vi "setState.vi"(0 "Interface in":T2, 7 "state":T1, 11 "error in (no error)":errorcluster) -> (4 "Interface out":T2, 15 "error out":errorcluster)   [LabVIEW 2017, in "BuckBoostInterface.lvlib"]
uses:
  BuckBoostInterface.lvlib
  Interface.ctl
  <instrlib>/_niInstr/Instruction Framework/v1/Host/Instruction Target/niInstr Instruction Target v1 Host.lvclass
  <instrlib>/_niInstr/Instruction Framework/v1/Host/Instruction Framework Context/niInstr Instruction Framework Context v1 Host.lvclass
  FPGA/contState.ctl
  <vilib>/NI/JSON Support for LabVIEW/JSON Data Classes/JSON Object/New JSON Object (Empty).vi
  <vilib>/NI/JSON Support for LabVIEW/JSON Data Classes/JSON Object/Insert Key Value Pair (Single).vi
  <vilib>/NI/JSON Support for LabVIEW/JSON Data Classes/JSON Helper/Parsing/Parse Value.vi
  <vilib>/NI/JSON Support for LabVIEW/JSON Data Classes/JSON Helper/To More Specific Type (Object).vi
  <vilib>/NI/JSON Support for LabVIEW/JSON Data Classes/JSON Datatype/JSON Null.lvclass
  <vilib>/NI/JSON Support for LabVIEW/JSON Data Classes/JSON Object/JSON Object.lvclass
  <vilib>/NI/JSON Support for LabVIEW/JSON Data Classes/JSON Helper/JSON Helper.lvclass
  FPGA/BuckBoost.lvlib
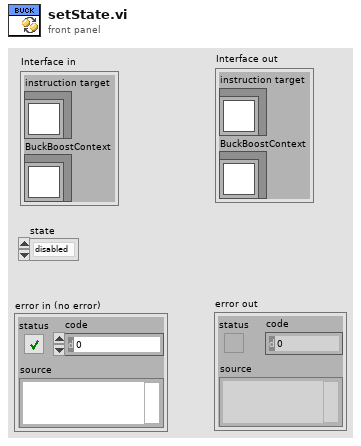
[diagram p1: front panel]
types:
  T1 = typedef "BuckBoost.lvlib/contState.ctl" = enum16{"disabled", "manual", "normal", "perturb"}
  T2 = typedef "BuckBoostInterface.lvlib/Interface.ctl" = cluster{"instruction target":refnum<class "niInstr Instruction Target v1 Host.lvclass">, "BuckBoostContext":refnum<class "niInstr Instruction Framework Context v1 Host.lvclass">}
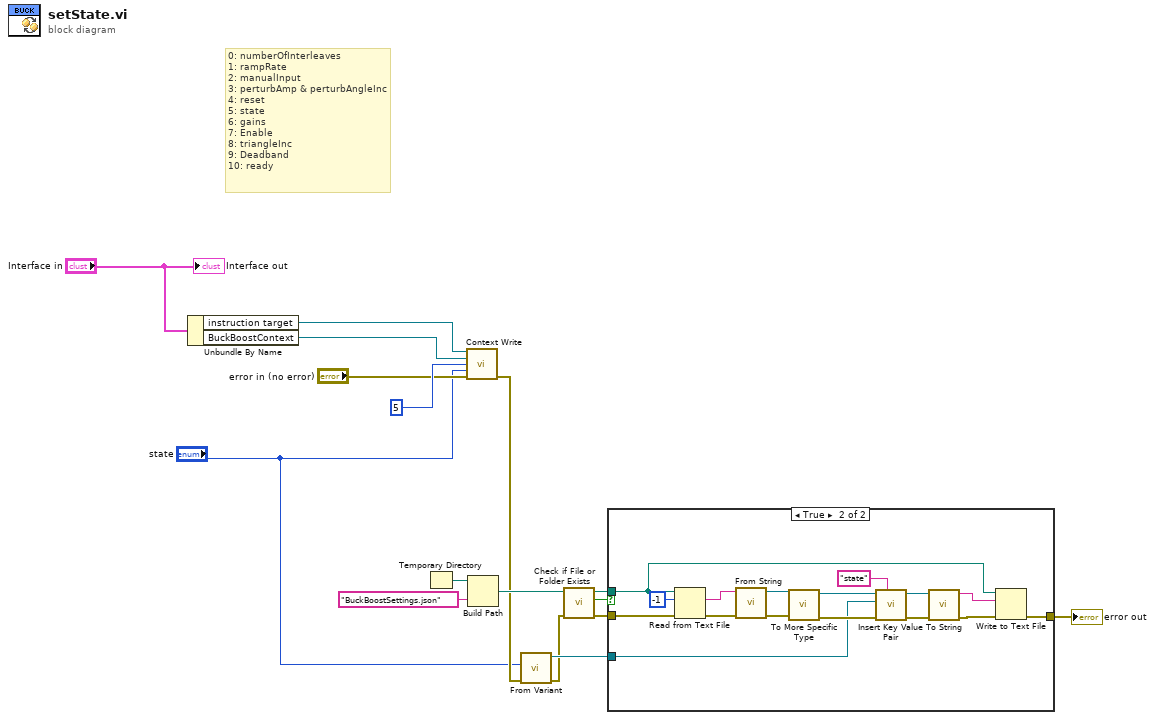
[diagram p0: block diagram]
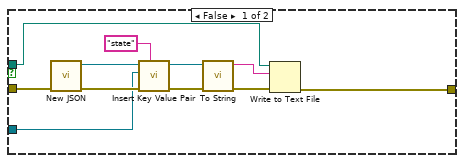
[diagram p2: hidden frame]
diagram:
  # "0: numberOfInterleaves\n1: rampRate\n2: manualInput\n3: perturbAmp & perturbAngleInc\n4: reset\n5: state\n6: gains\n7: Enable\n8: triangleInc\n9: Deadband\n10: ready"
  n1 = Unbundle By Name("Interface in") -> ("instruction target"=w13:refnum<class "niInstr Instruction Target v1 Host.lvclass">, "BuckBoostContext"=w12:refnum<class "niInstr Instruction Framework Context v1 Host.lvclass">)
  n2 = Temporary Directory() -> (w11:path)
  n3 = call <instrlib>:"Context Write.vi"("instruction target in"=w13, "context in"=w12, "address"=u64 5, "data"="state", "error in"="error in (no error)") -> ("error out"=w3:errorcluster)  [unwired: 8 in, 2 out]
  n4 = Build Path(base path=w11, name or relative path="BuckBoostSettings.json") -> (appended path=w9:path)
  n5 = call <vilib>:"From Variant.vi"("error in (no error)"=w3, "Variant"="state") -> ("error out"=w4:errorcluster, "JSON out"=w6:refnum<class "JSON Null.lvclass">)  [unwired: 8 in]
  n6 = call <vilib>:"Check if File or Folder Exists.vi"("error in (no error)"=w4, "path"=w9) -> ("error out"=w5:errorcluster, "file or folder exists?"=w7:bool, "dup path"=w8:path)  [unwired: 7 in]
  n7 = case shown="True" w7 {
    tunnel: w8 -> [w22 w34]
    tunnel: w6 -> [w24 w36]
    tunnel: w5 -> [w27 w35]
    tunnel: [w21 w29] -> w2
    frame False {
      n8 = call-poly <vilib>:"New JSON.vi"("error in (no error)"=w27) -> ("error out"=w25:errorcluster, "JSON Object out"=w26:refnum<class "JSON Object.lvclass">)  [unwired: 9 in]
      n9 = call-poly <vilib>:"Insert Key Value Pair.vi"("key"="state", "error in (no error)"=w25, "value"=w24, "JSON Object in"=w26) -> ("error out"=w20:errorcluster, "JSON Object out"=w17:refnum<class "JSON Object.lvclass">)  [unwired: 5 in, 1 out]
      n10 = call-dynamic "To String.vi"("error in (no error)"=w20, "JSON Object in"=w17) -> ("error out"=w19:errorcluster, "String"=w18:string)  [unwired: 8 in]
      n11 = Write to Text File(file (use dialog)=w22, text=w18, error in=w19) -> (error out=w21:errorcluster)  [unwired: 1 in, 2 out]
    }
    frame True {
      n12 = Read from Text File(file (use dialog)=w34, count=-1, error in=w35) -> (text=w43:string, error out=w38:errorcluster)  [unwired: 1 in, 2 out]
      n13 = call <vilib>:"From String.vi"("error in (no error)"=w38, "JSON String"=w43) -> ("error out"=w42:errorcluster, "JSON out"=w41:refnum<class "JSON Null.lvclass">)  [unwired: 8 in]
      n14 = call-poly <vilib>:"To More Specific Type.vi"("error in (no error)"=w42, "JSON Datatype in"=w41) -> ("error out"=w39:errorcluster, "JSON Datatype out"=w40:refnum<class "JSON Object.lvclass">)  [unwired: 8 in]
      n15 = call-poly <vilib>:"Insert Key Value Pair.vi"("key"="state", "error in (no error)"=w39, "value"=w36, "JSON Object in"=w40) -> ("error out"=w31:errorcluster, "JSON Object out"=w33:refnum<class "JSON Object.lvclass">)  [unwired: 5 in, 1 out]
      n16 = call-dynamic "To String.vi"("error in (no error)"=w31, "JSON Object in"=w33) -> ("error out"=w30:errorcluster, "String"=w32:string)  [unwired: 8 in]
      n17 = Write to Text File(file (use dialog)=w34, text=w32, error in=w30) -> (error out=w29:errorcluster)  [unwired: 1 in, 2 out]
    }
  }
  "error out" <- w2
  "Interface out" <- "Interface in"
